vi "AwtControllerModule.vi"() -> ()   [LabVIEW 2015]
uses:
  awt_modules.dll
panel:
  in  "DCFG \nIndex":string[][](table)=[["1"], ["2"], ["3"], ["4"], ["5"], ["6"], ["7"], ["8"], ["9"], ["10"], ["11"], ["12"], ["13"], ["14"], ["15"], ["16"], ["17"], ["18"], ["19"], ["20"], ["21"], ["22"], ["23"], ["24"], ["25"], ["26"]]
  out "UDP Response":string
  out "ReceivedResponse":u8[](array[numeric]) format="%x"
  in  "StopUDP":bool
  in  "Tab Control":T1(tab)
  in  "COM Port":u8=4
  in  "viewSel":i32=1
  in  "view":i32=1 min=1 max=3 step=1
  out "Reg Val (Hex)":u16 format="%x"
  in  "RegAddr (Hex)":i32=8 format="%x"
  in  "RegAddr (Hex)":i32 format="%x"
  in  "RegVal (Hex)":i32 format="%x"
  in  "logTransferEnable":bool=TRUE
  in  "udpTransferEnable":bool=TRUE
  in  "slot":i32=1 min=1 max=12 step=1
  in  "plot":i32=1 min=1 max=2 step=1
  in  "plotNo":i32=1 min=1 max=12 step=1
  in  "streamByte":i32=2
  in  "dcfgSel":i32
  in  "cloudDcfgSel":i32
  in  "CMD Selector":string(combo)
  in  "RxPort":i32=50002
  in  "TxPort":i32=50001
  # "Stop UDP before closing\n LabView Session"
  # "CMD ID"
  # "Status Byte"
  # "Status Byte\tDetails\n0x00\tSuccess\n0x01\tFailure\n0x04\tNo View Available\n0x05\tSensor is already in Play State\n0x06\tSensor in already in Stop State\n0x07\tNot in stop state\n0x09\tCommand is Not Applicable\n0x0A\tTarget board is already connected\n0x0B\tInvalid Command\n0x0C\tFailed to Open the View or View already opened\n0x0D\tFailed to Load the config file\n0x0E\tThe parameter entered is Invalid \n0x0F\tList the Views first and then use Open view command\n0xA0\tViews plugin removed or Not found\n0xB0\tNo Configuration file found\n0xC0\tTarget board is not connected \n0xE0\tConfig file not available\n0xF0\tOperation Failed. No Device connected\n0x11\tCommand is not supported \n0x12\tChannel selection failed, since sensor is in Play state\n0x13\tChannel is not enabled\n0x1A\tThe device is already disconnected\n0x1B\tLoad Config failed since sensor is in Play state\n0x1E\tCannot enable Raw data, already in On State\n0x1F\tCannot disable Raw data, already in Off State\n0x2A\tNo Config files loaded\n0x2B\tCannot enable Logging, already in On State\n0x2C\tCannot disable Logging, already in Off State\n0x2D\tThe Selected Slot is not enabled\n0x2E\tSlot select failed. Sensor is in Play State\n0x2F\tSoftware reset failed. Sensor is in Play State."
  # "Command\tResponse ID\nCONNECT           \t         0x99\nDISCONNECT        \t       0x91\nLIST_CONFIG                 0x95\nLOAD_CONFIG       \t      0x97\nLIST_CLOUD_CFG \t       0x98\nLOAD_CLOUD_CFG \t    0x9A\nREAD              \t                0x80\nWRITE             \t               0x081\nPLAY              \t                0x82\nSTOP                              \t0x83\nLIST_VIEW                       0x94\nOPEN_VIEW                    0x9E\nTAB_VIEW                      \t0x9C\nSLOT_SELECT                \t0x88\nCHANNEL_SELECT       \t0x9F\nSTREAM_RAWDATA    \t0x86\nSAVE_LOG                     \t0x85\nSOFTWARE_RESET       \t0x9B"
  # "ListView to be called before opening a view.\n\nList available in UDP Response and index starts at 1"
  # "1 - TimeView\n2- FrequencyView (ADPD 108)\n3 - Multislot View (ADPD 4xxx)"
  # "Bits order for selection\nOnly in Time View (ADPD 4xxx)\nS2 D2 S1 D1\n3   2   1    0  - (bits to be enabled)\nE.g. - S1 alone -> 2\nS1 and S2 -> 10"
  # "Call ListDcfg before Load\n\nListDcfg will give the available DCFG \nstarting from number 1 as index"
  # "Call ListCloudDcfg before Load\n\nListCloudDcfg will display the available DCFG \nstarting from number 1 as index in the UDP Response"
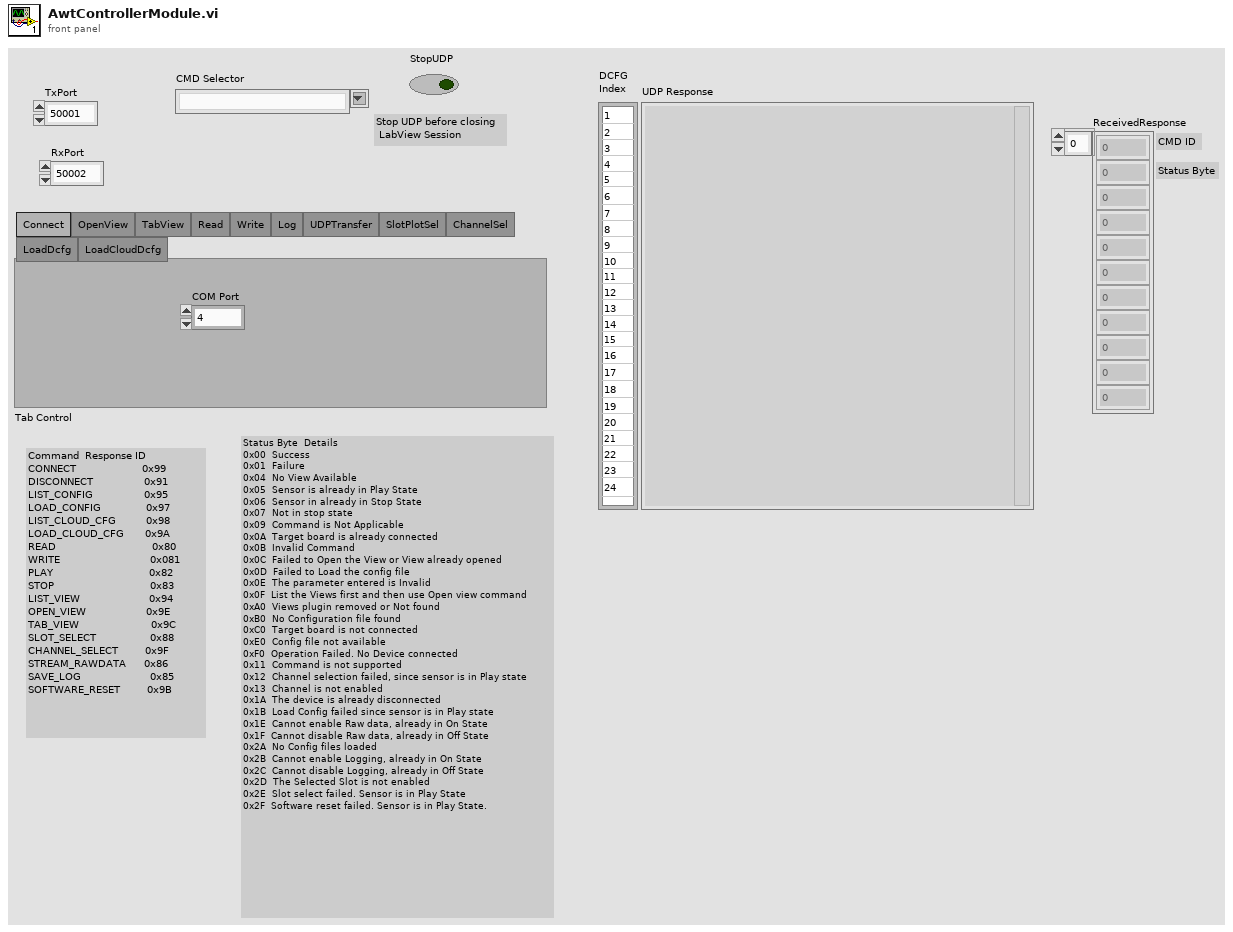
[diagram p1: front panel]
types:
  T1 = enum32{"Connect", "OpenView", "TabView", "Read", "Write", "Log", "UDPTransfer", "SlotPlotSel", "ChannelSel", "LoadDcfg", "LoadCloudDcfg"}
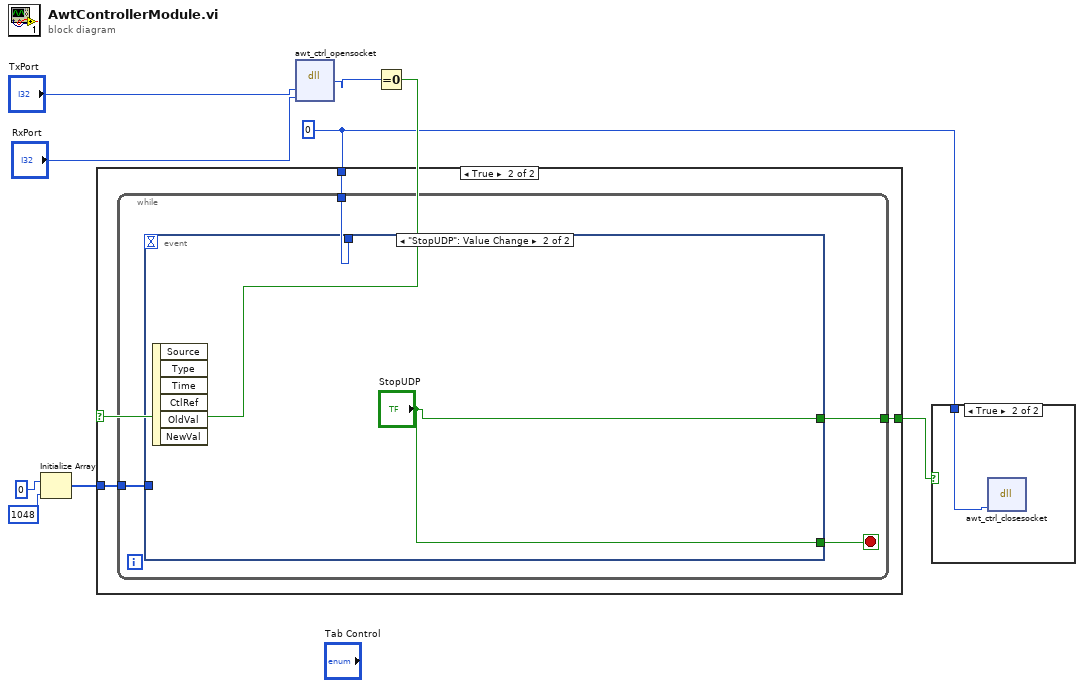
[diagram p0: block diagram]
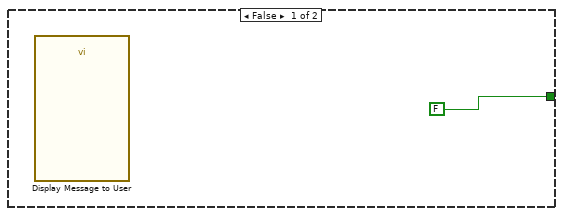
[diagram p3: hidden frame]
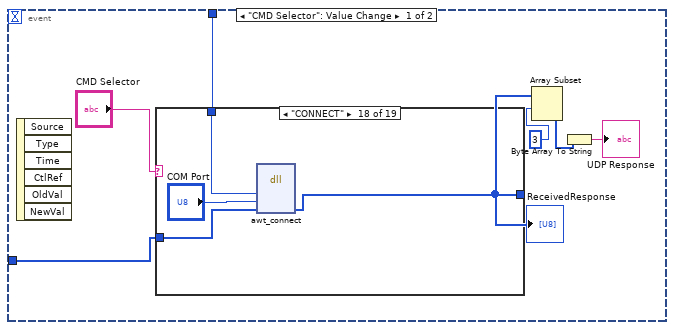
[diagram p4: hidden frame]
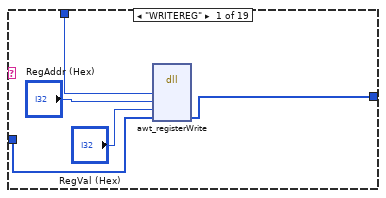
[diagram p5: hidden frame]
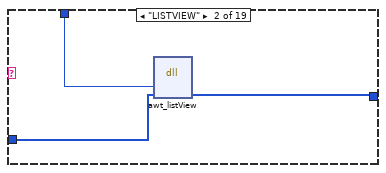
[diagram p6: hidden frame]
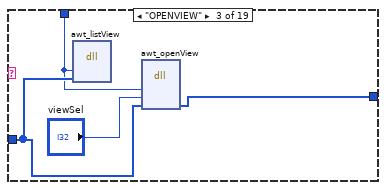
[diagram p7: hidden frame]
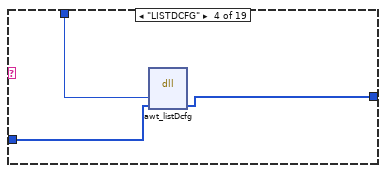
[diagram p8: hidden frame]
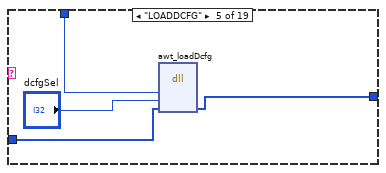
[diagram p9: hidden frame]
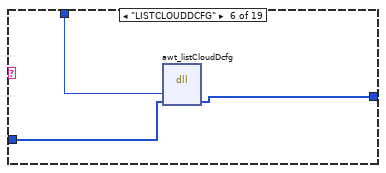
[diagram p10: hidden frame]
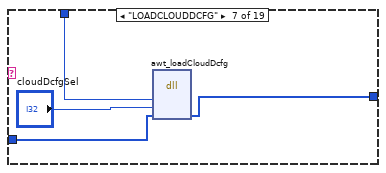
[diagram p11: hidden frame]
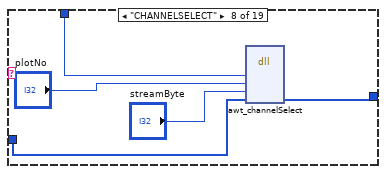
[diagram p12: hidden frame]
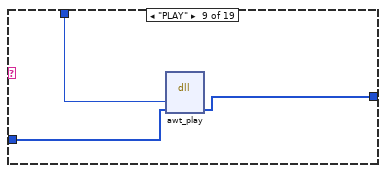
[diagram p13: hidden frame]
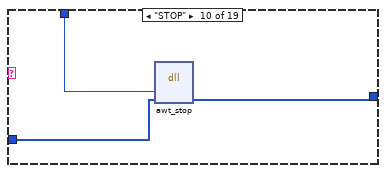
[diagram p14: hidden frame]
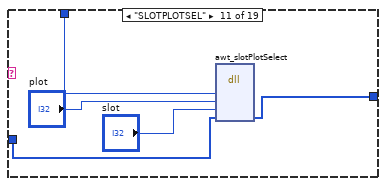
[diagram p15: hidden frame]
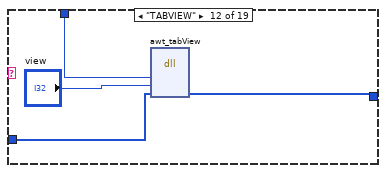
[diagram p16: hidden frame]
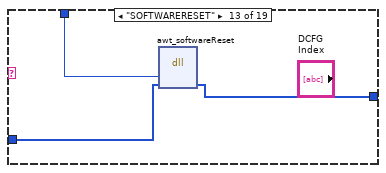
[diagram p17: hidden frame]
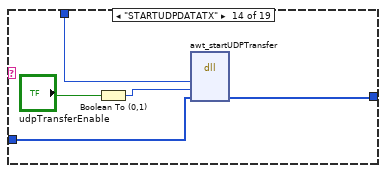
[diagram p18: hidden frame]
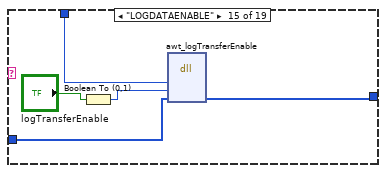
[diagram p19: hidden frame]
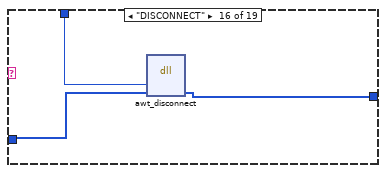
[diagram p20: hidden frame]
diagram:
  w1 = 0
  n1 = Initialize Array(u8 0, 1048) -> (w2:u8[])
  n2 = dll-call lib="C:/Users/ASIVAKUM/OneDrive - Analog Devices, Inc/Desktop/VSM/POC/UDP/Bidirectional_UDPmodules/UDP-Clib/AWT_LabView/awt_modules.dll" fn="awt_ctrl_opensocket"("txport"="TxPort", "rxport"="RxPort") -> ("return type"=w5:i32)  [unwired: 5 in, 2 out]
  n3 = Equal To 0?(x=w5) -> (x = 0?=w7:bool)
  n4 = case shown="True" w7 {
    tunnel: w1 -> [_ w13]
    tunnel: [FALSE w11] -> w6
    tunnel: w2 -> [_ w12]
    frame False {
      n5 = call "Display Message to User"() -> ()  [unwired: 10 in, 2 out]
    }
    frame True {
      n6 = while {
        tunnel: w13 -> [w17]
        tunnel: w12 -> [w16]
        tunnel: [w15] -> w11
        stop <- w14 stop-if-true
        n7 = event shown="[1] \"StopUDP\": Value Change" {
          selector: _ -> [_ _]
          dyn-events: _ -> [_ _]
          timeout: _ -> [_ _]
          tunnel: w17 -> [w23 _]
          tunnel: w16 -> [w21 _]
          tunnel: [_ "StopUDP"] -> w15
          tunnel: [_ "StopUDP"] -> w14
          event "CMD Selector": Value Change {
            n8 = event-data() -> ()  [unwired: 1 in, 6 out]
            n9 = case shown="\"CONNECT\"" "CMD Selector" {
              tunnel: w23 -> [w29 w32 w33 w37 w43 w46 w50 w55 w58 w61 w66 w70 w73 w78 w83 w86 _ w91 w98]
              tunnel: [w25 w30 w36 w38 w40 w44 w47 w51 w56 w59 w62 w67 w71 w76 w81 w84 w87 w88 w95] -> w20
              tunnel: w21 -> [w26 w31 w34 w39 w41 w45 w48 w52 w57 w60 w63 w68 w72 w77 w82 w85 w87 w90 w96]
              frame "WRITEREG" {
                n10 = dll-call lib="C:/Users/ASIVAKUM/OneDrive - Analog Devices, Inc/Desktop/VSM/POC/UDP/Bidirectional_UDPmodules/UDP-Clib/AWT_LabView/awt_modules.dll" fn="awt_registerWrite"("nInstId"=w29, "regAddr"="RegAddr (Hex)", "regVal"="RegVal (Hex)", "recvdBuf"=w26) -> ("recvdBuf"=w25:u8[])  [unwired: 7 in, 2 out]
              }
              frame "LISTVIEW" {
                n11 = dll-call lib="C:/Users/ASIVAKUM/OneDrive - Analog Devices, Inc/Desktop/VSM/POC/UDP/Bidirectional_UDPmodules/UDP-Clib/AWT_LabView/awt_modules.dll" fn="awt_listView"("nInstId"=w32, "recvdBuf"=w31) -> ("recvdBuf"=w30:u8[])  [unwired: 5 in, 2 out]
              }
              frame "OPENVIEW" {
                n12 = dll-call lib="C:/Users/ASIVAKUM/OneDrive - Analog Devices, Inc/Desktop/VSM/POC/UDP/Bidirectional_UDPmodules/UDP-Clib/AWT_LabView/awt_modules.dll" fn="awt_listView"("nInstId"=w33, "recvdBuf"=w34) -> ()  [unwired: 6 in, 2 out]
                n13 = dll-call lib="C:/Users/ASIVAKUM/OneDrive - Analog Devices, Inc/Desktop/VSM/POC/UDP/Bidirectional_UDPmodules/UDP-Clib/AWT_LabView/awt_modules.dll" fn="awt_openView"("nInstId"=w33, "viewSel"="viewSel", "recvdBuf"=w34) -> ("recvdBuf"=w36:u8[])  [unwired: 6 in, 2 out]
              }
              frame "LISTDCFG" {
                n14 = dll-call lib="C:/Users/ASIVAKUM/OneDrive - Analog Devices, Inc/Desktop/VSM/POC/UDP/Bidirectional_UDPmodules/UDP-Clib/AWT_LabView/awt_modules.dll" fn="awt_listDcfg"("nInstId"=w37, "recvdBuf"=w39) -> ("recvdBuf"=w38:u8[])  [unwired: 5 in, 2 out]
              }
              frame "LOADDCFG" {
                n15 = dll-call lib="C:/Users/ASIVAKUM/OneDrive - Analog Devices, Inc/Desktop/VSM/POC/UDP/Bidirectional_UDPmodules/UDP-Clib/AWT_LabView/awt_modules.dll" fn="awt_loadDcfg"("nInstId"=w43, "dcfgSel"="dcfgSel", "recvdBuf"=w41) -> ("recvdBuf"=w40:u8[])  [unwired: 6 in, 2 out]
              }
              frame "LISTCLOUDDCFG" {
                n16 = dll-call lib="C:/Users/ASIVAKUM/OneDrive - Analog Devices, Inc/Desktop/VSM/POC/UDP/Bidirectional_UDPmodules/UDP-Clib/AWT_LabView/awt_modules.dll" fn="awt_listCloudDcfg"("nInstId"=w46, "recvdBuf"=w45) -> ("recvdBuf"=w44:u8[])  [unwired: 5 in, 2 out]
              }
              frame "LOADCLOUDDCFG" {
                n17 = dll-call lib="C:/Users/ASIVAKUM/OneDrive - Analog Devices, Inc/Desktop/VSM/POC/UDP/Bidirectional_UDPmodules/UDP-Clib/AWT_LabView/awt_modules.dll" fn="awt_loadCloudDcfg"("nInstId"=w50, "cloudDcfgSel"="cloudDcfgSel", "recvdBuf"=w48) -> ("recvdBuf"=w47:u8[])  [unwired: 6 in, 2 out]
              }
              frame "CHANNELSELECT" {
                n18 = dll-call lib="C:/Users/ASIVAKUM/OneDrive - Analog Devices, Inc/Desktop/VSM/POC/UDP/Bidirectional_UDPmodules/UDP-Clib/AWT_LabView/awt_modules.dll" fn="awt_channelSelect"("nInstId"=w55, "plotNo"="plotNo", "streamByte"="streamByte", "recvdBuf"=w52) -> ("recvdBuf"=w51:u8[])  [unwired: 7 in, 2 out]
              }
              frame "PLAY" {
                n19 = dll-call lib="C:/Users/ASIVAKUM/OneDrive - Analog Devices, Inc/Desktop/VSM/POC/UDP/Bidirectional_UDPmodules/UDP-Clib/AWT_LabView/awt_modules.dll" fn="awt_play"("nInstId"=w58, "recvdBuf"=w57) -> ("recvdBuf"=w56:u8[])  [unwired: 5 in, 2 out]
              }
              frame "STOP" {
                n20 = dll-call lib="C:/Users/ASIVAKUM/OneDrive - Analog Devices, Inc/Desktop/VSM/POC/UDP/Bidirectional_UDPmodules/UDP-Clib/AWT_LabView/awt_modules.dll" fn="awt_stop"("nInstId"=w61, "recvdBuf"=w60) -> ("recvdBuf"=w59:u8[])  [unwired: 5 in, 2 out]
              }
              frame "SLOTPLOTSEL" {
                n21 = dll-call lib="C:/Users/ASIVAKUM/OneDrive - Analog Devices, Inc/Desktop/VSM/POC/UDP/Bidirectional_UDPmodules/UDP-Clib/AWT_LabView/awt_modules.dll" fn="awt_slotPlotSelect"("nInstId"=w66, "plot"="plot", "slot"="slot", "recvdBuf"=w63) -> ("recvdBuf"=w62:u8[])  [unwired: 7 in, 2 out]
              }
              frame "TABVIEW" {
                n22 = dll-call lib="C:/Users/ASIVAKUM/OneDrive - Analog Devices, Inc/Desktop/VSM/POC/UDP/Bidirectional_UDPmodules/UDP-Clib/AWT_LabView/awt_modules.dll" fn="awt_tabView"("nInstId"=w70, "view"="view", "recvdBuf"=w68) -> ("recvdBuf"=w67:u8[])  [unwired: 6 in, 2 out]
              }
              frame "SOFTWARERESET" {
                n23 = dll-call lib="C:/Users/ASIVAKUM/OneDrive - Analog Devices, Inc/Desktop/VSM/POC/UDP/Bidirectional_UDPmodules/UDP-Clib/AWT_LabView/awt_modules.dll" fn="awt_softwareReset"("nInstId"=w73, "recvdBuf"=w72) -> ("recvdBuf"=w71:u8[])  [unwired: 5 in, 2 out]
              }
              frame "STARTUDPDATATX" {
                n24 = Boolean To (0,1)(Boolean="udpTransferEnable") -> (0, 1=w74:i16)
                n25 = dll-call lib="C:/Users/ASIVAKUM/OneDrive - Analog Devices, Inc/Desktop/VSM/POC/UDP/Bidirectional_UDPmodules/UDP-Clib/AWT_LabView/awt_modules.dll" fn="awt_startUDPTransfer"("nInstId"=w78, "udpTransferEnable"=w74, "recvdBuf"=w77) -> ("recvdBuf"=w76:u8[])  [unwired: 6 in, 2 out]
              }
              frame "LOGDATAENABLE" {
                n26 = Boolean To (0,1)(Boolean="logTransferEnable") -> (0, 1=w79:i16)
                n27 = dll-call lib="C:/Users/ASIVAKUM/OneDrive - Analog Devices, Inc/Desktop/VSM/POC/UDP/Bidirectional_UDPmodules/UDP-Clib/AWT_LabView/awt_modules.dll" fn="awt_logTransferEnable"("nInstId"=w83, "logTransferEnable"=w79, "recvdBuf"=w82) -> ("recvdBuf"=w81:u8[])  [unwired: 6 in, 2 out]
              }
              frame "DISCONNECT" {
                n28 = dll-call lib="C:/Users/ASIVAKUM/OneDrive - Analog Devices, Inc/Desktop/VSM/POC/UDP/Bidirectional_UDPmodules/UDP-Clib/AWT_LabView/awt_modules.dll" fn="awt_disconnect"("nInstId"=w86, "recvdBuf"=w85) -> ("recvdBuf"=w84:u8[])  [unwired: 5 in, 2 out]
              }
              frame Default {
              }
              frame "CONNECT" {
                n29 = dll-call lib="C:/Users/ASIVAKUM/OneDrive - Analog Devices, Inc/Desktop/VSM/POC/UDP/Bidirectional_UDPmodules/UDP-Clib/AWT_LabView/awt_modules.dll" fn="awt_connect"("nInstId"=w91, "portNum"="COM Port", "recvdBuf"=w90) -> ("recvdBuf"=w88:u8[])  [unwired: 6 in, 2 out]
              }
              frame "READREG" {
                n30 = dll-call lib="C:/Users/ASIVAKUM/OneDrive - Analog Devices, Inc/Desktop/VSM/POC/UDP/Bidirectional_UDPmodules/UDP-Clib/AWT_LabView/awt_modules.dll" fn="awt_registerRead"("nInstId"=w98, "regAddr"="RegAddr (Hex)", "recvdBuf"=w96, "pRegVal"=u16 0) -> ("recvdBuf"=w95:u8[], "pRegVal"=→"Reg Val (Hex)":u16)  [unwired: 6 in, 2 out]
                n31 = Index Array(array=w95, index=3) -> ()  [unwired: 1 out]
              }
            }
            "ReceivedResponse" <- w20
            n32 = Array Subset(array=w20, index=3) -> (w18:u8[])  [unwired: 1 in]
            n33 = Byte Array To String(unsigned byte array=w18) -> (string=→"UDP Response":string)
          }
          event "StopUDP": Value Change {
            n34 = event-data() -> ()  [unwired: 1 in, 6 out]
          }
        }
      }
    }
  }
  n35 = case shown="True" w6 {
    tunnel: w1 -> [_ w100]
    frame False {
    }
    frame True {
      n36 = dll-call lib="C:/Users/ASIVAKUM/OneDrive - Analog Devices, Inc/Desktop/VSM/POC/UDP/Bidirectional_UDPmodules/UDP-Clib/AWT_LabView/awt_modules.dll" fn="awt_ctrl_closesocket"("nInstId"=w100) -> ()  [unwired: 5 in, 2 out]
    }
  }
